vi "Robot Global Data.vi"() -> ()   [LabVIEW 2018]
doc: "This global VI can contain as many global variables as you need. Place a control on the panel, give it a good name. To read or write to it from a VI, drag the icon to the diagram of that VI. You can also drag from the project. Click on the node to change which global you access. You shouldn't have multiple locations writing to a global or it will cause a race-condition."
uses:
  <vilib>/Rock Robotics/WPI/Camera/WPI_CameraImageSize.ctl
  <vilib>/Rock Robotics/WPI/DriverStation/WPI_DriverStationRobotMode2.ctl
panel:
  in  "ejectHatch":bool
  out "startIntakeTime":timestamp
  out "desiredForebarVal":dbl
  out "desiredDorsalVal":dbl
  in  "reqTest":bool
  in  "reqShootPos":bool
  in  "reqGround":bool
  in  "reqHover":bool
  in  "reqPosHatch":bool
  in  "reqHome":bool
  out "shoot":bool
  out "intake":bool
  in  "maxMotorSpeed":dbl
  in  "forebarShootAngle":dbl
  in  "dorsalShootAngle":dbl
  out "forebarPotVal":dbl
  out "dorsalPotVal":dbl
  out "dorsalDown":bool
  out "cargo":bool
  out "lineCentOn":bool
  out "lineRightOn":bool
  out "lineLeftOn":bool
  out "forebarBack":bool
  out "forebarFwd":bool
  out "dorsalUp":bool
  in  "Gyro Reset Deltas?":bool
  out "IMU Angle Delta":cluster{"X":dbl, "Y":dbl, "Z":dbl}
  out "Gyro Sensor Ready?":bool
  out "IMU Data":T1
  in  "Robot Mode":T2
  in  "image size":T3=enum."320x240"
  in  "Enable Vision":bool
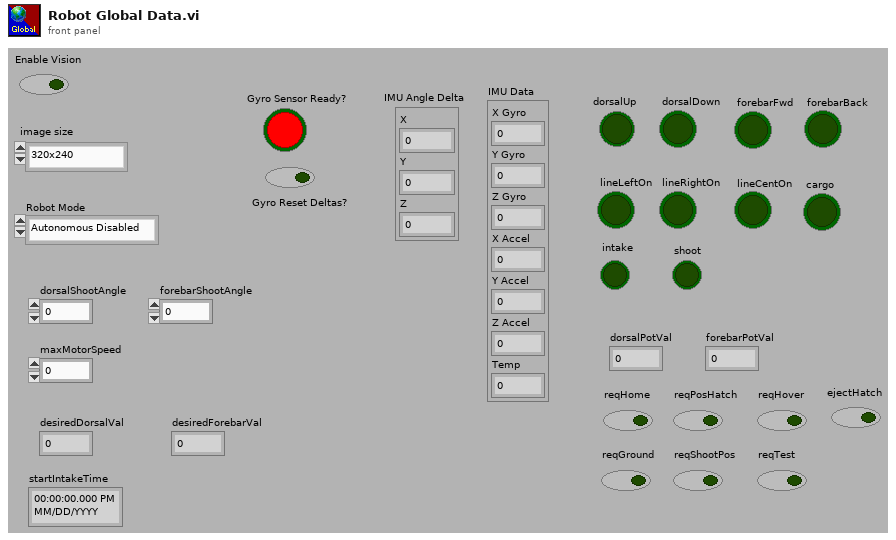
[diagram p1: front panel]
types:
  T1 = cluster{"X Gyro":dbl, "Y Gyro":dbl, "Z Gyro":dbl, "X Accel":dbl, "Y Accel":dbl, "Z Accel":dbl, "Temp":dbl}
  T2 = typedef "WPI_DriverStationRobotMode2.ctl" = enum16{"Autonomous Disabled", "Autonomous Enabled", "Teleop Disabled", "Teleop Enabled", "Disconnected", "Finish", "Test Disabled", "Test Enabled", "Emergency Stopped"}
  T3 = typedef "WPI_CameraImageSize.ctl" = enum16{"640x480", "320x240", "160x120", "Custom"}
diagram:
